vi "Queue_WaitForResponse.vi"(8 "error in (no error)":errorcluster, 9 "QueueTimeout_ms (10000)":i32, 10 "CloseQueue [T]":bool=TRUE, 11 "Response Queue":refnum<queue>) -> (0 "error out":errorcluster, 1 "HttpContent out":refnum<class "HttpContent.lvclass">, 2 "HTTPHeaders_NET out":refnum<class "HttpHeaders_Response.lvclass">, 3 "HttpResponseMessage out":refnum<class "HttpResponseMessage.lvclass">, 4 "Queue timed out?":bool, 5 "StatusCode":i32, 6 "ReasonPhrase":string, 7 "TaskSuccess":bool)   [LabVIEW 2018, in "HttpClient_NET.lvlib" / "HttpClient_NET.lvclass"]
doc: "<b> </b> <b> </b>\nHttpClient_NET\nJustin Young - Viviota\nCopyright (c) 2021\nLicense: BSD"
uses:
  HttpClient_NET.lvclass
  HttpResponseMessage/HttpResponseMessage.lvclass
  HttpResponseMessage/Types/ResponseMessage_Cluster.ctl
  HttpContent/HttpContent.lvclass
  HttpHeaders_response/HttpHeaders_Response.lvclass
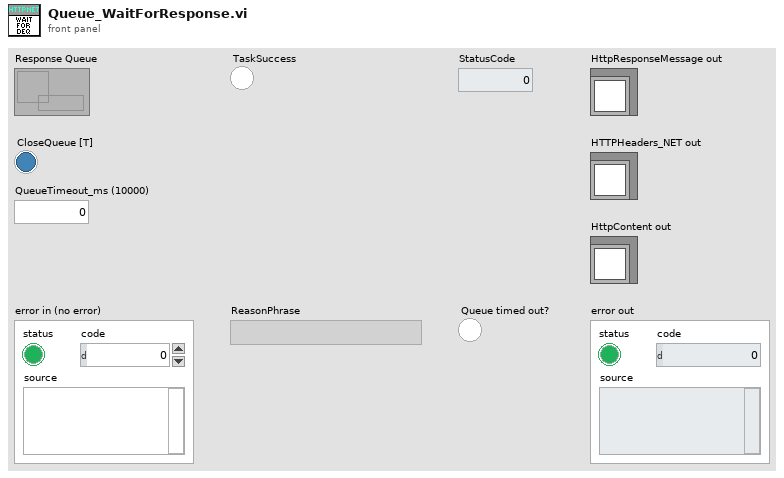
[diagram p1: front panel]
types:
  T1 = typedef "HttpClient_NET.lvlib/HttpResponseMessage.lvclass/ResponseMessage_Cluster.ctl" = cluster{"HttpResponseMessage":refnum<class "HttpResponseMessage.lvclass">, "TaskSuccess":bool}
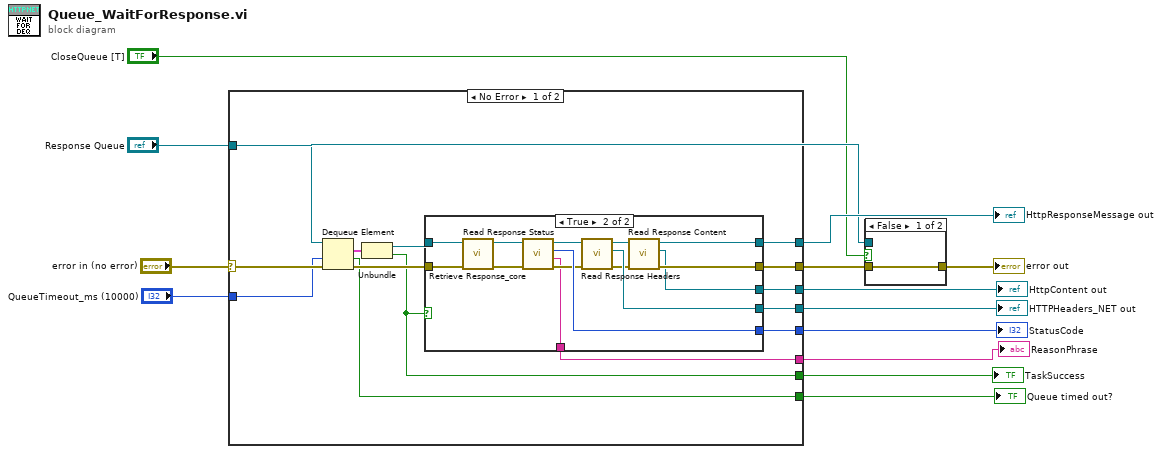
[diagram p0: block diagram]
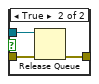
[diagram p4: hidden frame]
diagram:
  n1 = case shown="No Error" "error in (no error)" {
    selector: "error in (no error)" -> [w27 w44]
    tunnel: [w26 _] -> w12
    tunnel: [w25 w44] -> w11
    tunnel: [w23 _] -> w10
    tunnel: [w20 _] -> w9
    tunnel: [w19 _] -> w8
    tunnel: [w18 _] -> w7
    tunnel: "QueueTimeout_ms (10000)" -> [w17 _]
    tunnel: [w16 _] -> w5
    tunnel: "Response Queue" -> [w15 _]
    tunnel: [w14 _] -> w1
    frame No Error {
      n2 = Dequeue Element(queue=w15, timeout in ms (-1)=w17, error in (no error)=w27) -> (element=w21:T1, timed out?=w16:bool, error out=w24:errorcluster)  [unwired: 1 out]
      n3 = Unbundle(w21) -> ("HttpResponseMessage"=w22:refnum<class "HttpResponseMessage.lvclass">, "TaskSuccess"=w23:bool)
      n4 = case shown="True" w23 {
        tunnel: [w28 w43] -> w25
        tunnel: [_ w42] -> w18
        tunnel: [w29 w41] -> w26
        tunnel: [_ w40] -> w19
        tunnel: [_ w39] -> w20
        tunnel: w24 -> [w28 w32]
        tunnel: w22 -> [w29 w33]
        tunnel: [_ w34] -> w14
        frame False {
        }
        frame True {
          n5 = call "Retrieve Response_core.vi"("error in (no error)"=w32, "HttpResponseMessage in"=w33) -> ("error out"=w31:errorcluster, "HttpResponseMessage out"=w30:refnum<class "HttpResponseMessage.lvclass">)  [unwired: 6 in, 2 out]
          n6 = call "Read Response Status.vi"("error in (no error)"=w31, "HttpResponseMessage in"=w30) -> ("error out"=w36:errorcluster, "ReasonPhrase"=w34:string, "StatusCode"=w42:i32, "HttpResponseMessage out"=w35:refnum<class "HttpResponseMessage.lvclass">)  [unwired: 4 in, 2 out]
          n7 = call "Read Response Headers.vi"("error in (no error)"=w36, "HttpResponseMessage in"=w35) -> ("error out"=w38:errorcluster, "HTTPHeaders_NET out"=w40:refnum<class "HttpHeaders_Response.lvclass">, "HttpResponseMessage out"=w37:refnum<class "HttpResponseMessage.lvclass">)  [unwired: 7 in]
          n8 = call "Read Response Content.vi"("error in (no error)"=w38, "HttpResponseMessage in"=w37) -> ("error out"=w43:errorcluster, "HttpContent out"=w39:refnum<class "HttpContent.lvclass">, "HttpResponseMessage out"=w41:refnum<class "HttpResponseMessage.lvclass">)  [unwired: 7 in]
        }
      }
    }
    frame Error {
    }
  }
  "HttpResponseMessage out" <- w12
  "HttpContent out" <- w9
  "HTTPHeaders_NET out" <- w8
  "StatusCode" <- w7
  "TaskSuccess" <- w10
  "Queue timed out?" <- w5
  "ReasonPhrase" <- w1
  n9 = case shown="False" "CloseQueue [T]" {
    tunnel: w11 -> [w45 w48]
    tunnel: [w45 w47] -> w4
    tunnel: "Response Queue" -> [_ w46]
    frame False {
    }
    frame True {
      n10 = Release Queue(queue=w46, error in (no error)=w48) -> (error out=w47:errorcluster)  [unwired: 1 in, 2 out]
    }
  }
  "error out" <- w4
